vi "2023 Create CVS Control Spreadsheet.vi"(0 "error in":errorcluster) -> (1 "localControlSpreadSheet":string[][](array[string]), 2 "error out":errorcluster)   [LabVIEW 2020]
uses:
  <vilib>/Utility/file.llb/Read Delimited Spreadsheet (string).vi
  SpreadSheetGlobal.vi
panel:
  in  "file path for Win":path=path "C:/git/981LabViewComponents/ControlSpreadsheet.csv"
  in  "file path for linux":path=path "/home/lvuser/ControlSpreadsheet.csv"
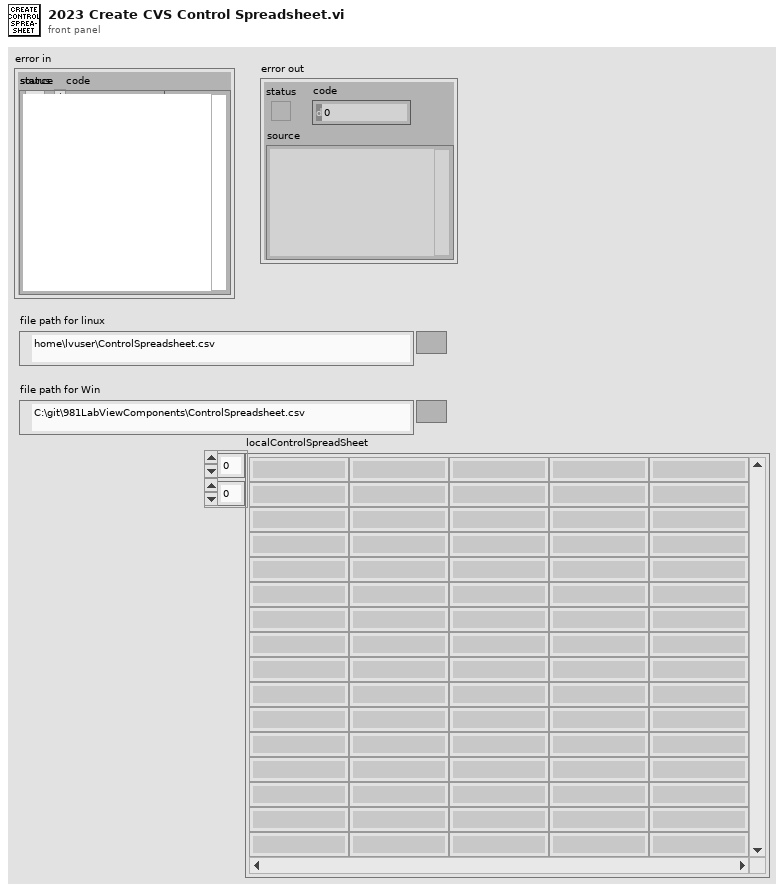
[diagram p1: front panel]
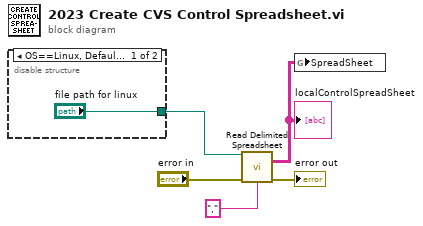
[diagram p0: block diagram]
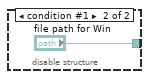
[diagram p2: hidden frame]
diagram:
  n1 = disable-structure shown="OS==Linux, Default" {
    disable-tunnel: ["file path for linux" "file path for Win"] -> w3
    frame condition #0 (active) {
    }
    frame condition #1 {
    }
  }
  n2 = call-poly <vilib>:"Read Delimited Spreadsheet.vi"("file path (dialog if empty)"=w3, "error in (no error)"="error in", "delimiter (\\t)"="," ("delimiter (\\t)")) -> ("all rows"=w1:string[][], "error out"=→"error out":errorcluster)  [unwired: 7 in, 4 out]
  "localControlSpreadSheet" <- w1
  n3 = global write "SpreadSheetGlobal.vi" "SpreadSheet"(w1) -> ()
